vi "Decide next action (polarization-based).vi"(8 "error in (no error)":errorcluster, 10 "Seek positive polarization?":bool, 11 "Automation in":refnum<class "Automation.lvclass">) -> (0 "error out":errorcluster, 1 "Should reseek?":bool, 2 "Decision":T1, 3 "Automation out":refnum<class "Automation.lvclass">)   [LabVIEW 2019, in "Automation.lvclass"]
uses:
  Automation.lvclass
  Automatic mode/Controller decision.ctl
  Automation.lvclass/Automation.ctl
  <vilib>/Analysis/baseanly.llb/Mean (DBL).vi
  <vilib>/Analysis/NI_AALBase.lvlib
  <vilib>/gmath/NI_Gmath.lvlib
panel:
  out "Polarizations":dbl[](array[numeric])
  out "mean":dbl format="%0.2f"
  out "Last polarization":dbl
  out "spread value":dbl
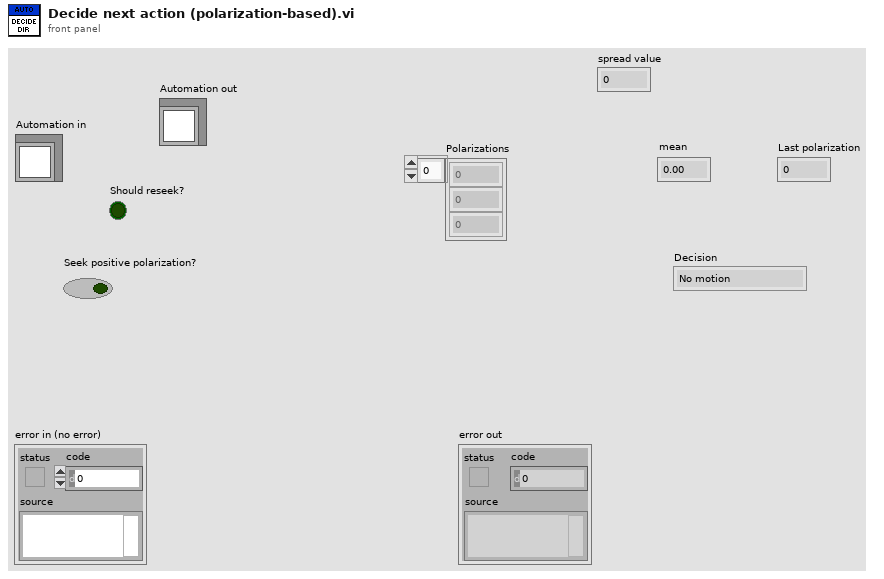
[diagram p1: front panel]
types:
  T1 = typedef "Controller decision.ctl" = enum16{"No motion", "Switch direction", "Keep current direction"}
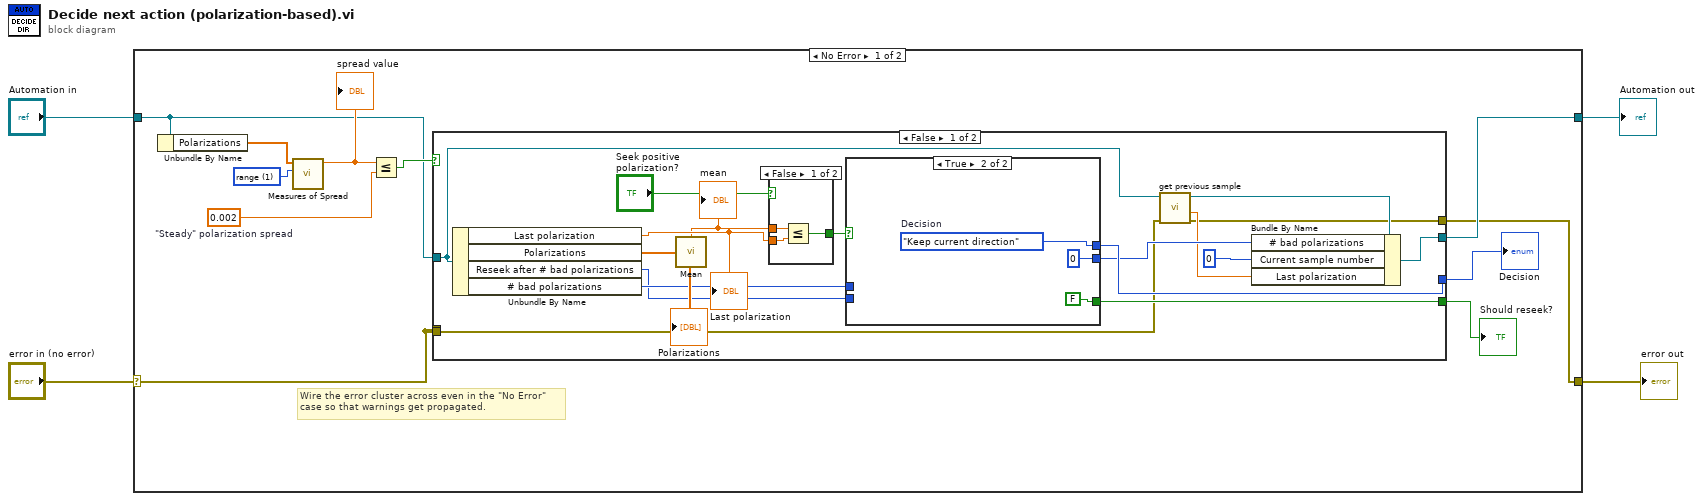
[diagram p0: block diagram]
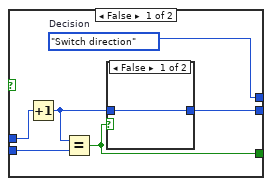
[diagram p2: hidden frame]
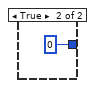
[diagram p3: hidden frame]
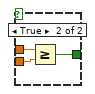
[diagram p4: hidden frame]
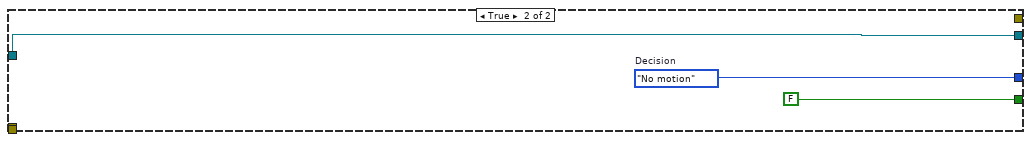
[diagram p5: hidden frame]
diagram:
  n1 = case shown="No Error" "error in (no error)" {
    selector: "error in (no error)" -> [w5 w54]
    tunnel: [w6 w54] -> w3
    tunnel: [w9 w53] -> w1
    tunnel: "Automation in" -> [w11 w53]
    frame No Error {
      w13 = 0.002  # "Steady" polarization spread
      w15 = 1 items=["standard deviation", "range", "mean absolute deviation", "interquartile range"] ("type")
      # "Wire the error cluster across even in the \"No Error\"\ncase so that warnings get propagated."
      n2 = Unbundle By Name(w11) -> ("Polarizations"=w10:dbl[])
      n3 = call <vilib>:"Measures of Spread.vi"("type"=w15, "x array"=w10) -> ("spread value"=w14:dbl)  [unwired: 8 in, 1 out]
      "spread value" <- w14
      n4 = Less Or Equal?(x=w14, y=w13) -> (x <= y?=w12:bool)
      n5 = case shown="False" w12 {
        tunnel: [w23 w51] -> w9
        tunnel: [w29 w50] -> w8
        tunnel: [w24 FALSE] -> w7
        tunnel: w11 -> [w20 w51]
        tunnel: [w17 _] -> w6
        tunnel: w5 -> [_ _]
        tunnel: w5 -> [w16 _]
        frame False {
          n6 = Unbundle By Name(w20) -> ("Last polarization"=w31:dbl, "Polarizations"=w28:dbl[], "Reseek after # bad polarizations"=w22:u32, "# bad polarizations"=w25:u32)
          "Last polarization" <- w31
          "Polarizations" <- w28
          n7 = call-poly <vilib>:"Mean.vi"("X"=w28) -> ("mean"=w27:dbl)  [unwired: 1 out]
          "mean" <- w27
          n8 = case shown="False" "Seek positive polarization?" {
            tunnel: w27 -> [w46 w49]
            tunnel: w31 -> [w45 w48]
            tunnel: [w44 w47] -> w30
            frame False {
              n9 = Less Or Equal?(x=w46, y=w45) -> (x <= y?=w44:bool)
            }
            frame True {
              n10 = Greater Or Equal?(x=w49, y=w48) -> (x >= y?=w47:bool)
            }
          }
          n11 = case shown="True" w30 {
            tunnel: [w33 w41] -> w29
            tunnel: [w35 u32 0] -> w26
            tunnel: w25 -> [w38 _]
            tunnel: [w36 FALSE] -> w24
            tunnel: w22 -> [w37 _]
            frame False {
              w33 = Controller_decision."Switch direction"  # Decision
              n12 = Increment(x=w38) -> (x+1=w34:u32)
              n13 = Equal?(x=w34, y=w37) -> (x = y?=w36:bool)
              n14 = case shown="False" w36 {
                tunnel: [w39 0] -> w35
                tunnel: w34 -> [w39 _]
                frame False {
                }
                frame True {
                }
              }
            }
            frame True {
              w41 = Controller_decision."Keep current direction"  # Decision
            }
          }
          n15 = call "get previous sample.vi"("error in (no error)"=w16, "Automation in"=w20) -> ("error out"=w17:errorcluster, "Polarization"=w18:dbl, "Automation out"=w19:refnum<class "Automation.lvclass">)  [unwired: 6 in, 1 out]
          n16 = Bundle By Name(cluster=w19, "# bad polarizations"=w26, "Current sample number"=0, "Last polarization"=w18) -> (w23:refnum<class "Automation.lvclass">)
        }
        frame True {
          w50 = Controller_decision."No motion"  # Decision
        }
      }
      "Decision" <- w8
      "Should reseek?" <- w7
    }
    frame Error {
    }
  }
  "error out" <- w3
  "Automation out" <- w1
